vi "Wait for Operation Complete.vi"(8 "error in (no error)":errorcluster, 9 "Maximum Time (10000ms)":i32=10000, 11 "VISA resource name":refnum<visa-resource-name>) -> (0 "error out":errorcluster, 3 "VISA resource name out":refnum<visa-resource-name>)   [LabVIEW 2014, in "Agilent ESA PSA Series.lvlib"]
doc: "Waits for the current operation to finish. This VI should be called after Initiate VI.\n\n<B>Note:</B> \n\nUse this VI only with other low-level VIs. The high-level VIs automatically incorporate this functionality. This VI does not check the instrument status."
uses:
  Agilent ESA PSA Series.lvlib
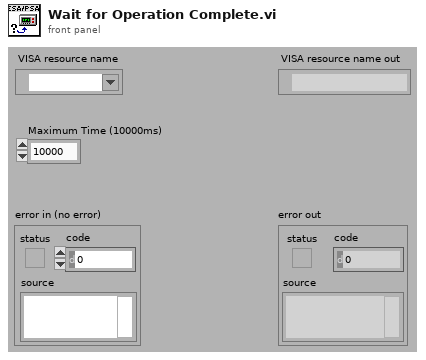
[diagram p1: front panel]
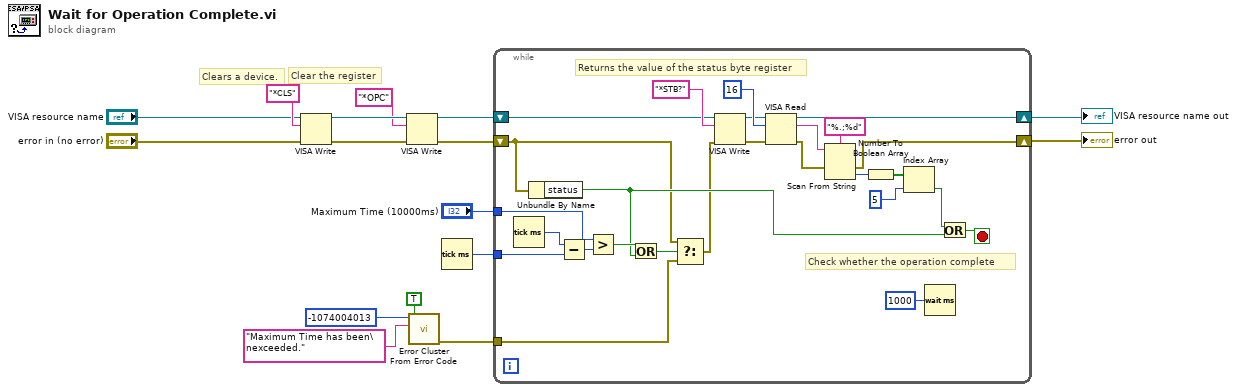
[diagram p0: block diagram]
diagram:
  # "Clears a device."
  # "Clear the register"
  n1 = VISA Write(VISA resource name="VISA resource name", write buffer="*CLS", error in (no error)="error in (no error)") -> (VISA resource name out=w6:refnum<visa-resource-name>, error out=w7:errorcluster)  [unwired: 1 out]
  n2 = VISA Write(VISA resource name=w6, write buffer="*OPC", error in (no error)=w7) -> (VISA resource name out=w5:refnum<visa-resource-name>, error out=w4:errorcluster)  [unwired: 1 out]
  n3 = call "Error Cluster From Error Code.vi"("show call chain? (False)"=TRUE, "error message (\"\")"="Maximum Time has been\nexceeded." ("error message (\"\")"), "error code (0)"=-1074004013) -> ("error out"=w10:errorcluster)  [unwired: 6 in]
  n4 = Tick Count (ms)() -> (millisecond timer value=w15:u32)
  n5 = while {
    tunnel: "Maximum Time (10000ms)" -> [w25]
    tunnel: w15 -> [w33]
    tunnel: w10 -> [w20]
    shift-right: [w31] -> w8
    shift-left: w4 -> [w18]
    shift-right: [w40] -> w9
    shift-left: w5 -> [w37]
    stop <- w26 stop-if-true
    # "Check whether the operation complete"
    # "Returns the value of the status byte register"
    n6 = Tick Count (ms)() -> (millisecond timer value=w34:u32)
    n7 = Unbundle By Name(w18) -> ("status"=w21:bool)
    n8 = Subtract(x=w34, y=w33) -> (x-y=w24:u32)
    n9 = Greater?(x=w25, y=w24) -> (0:w23:bool)
    n10 = Or(x=w23, y=w21) -> (x .or. y?=w22:bool)
    n11 = Select(t=w18, s=w22, f=w20) -> (s? t:f=w19:errorcluster)
    n12 = VISA Write(VISA resource name=w37, write buffer="*STB?", error in (no error)=w19) -> (VISA resource name out=w35:refnum<visa-resource-name>, error out=w36:errorcluster)  [unwired: 1 out]
    n13 = VISA Read(VISA resource name=w35, byte count=u32 16, error in (no error)=w36) -> (VISA resource name out=w40:refnum<visa-resource-name>, read buffer=w42:string, error out=w32:errorcluster)  [unwired: 1 out]
    n14 = Scan From String(format string="%.;%d", input string=w42, error in=w32) -> (error out=w31:errorcluster, output 1=w28:i32)  [unwired: 2 in, 2 out]
    n15 = Number To Boolean Array(number=w28) -> (Boolean array=w29:bool[])
    n16 = Index Array(array=w29, index=5) -> (element=w27:bool)
    n17 = Wait (ms)(milliseconds to wait=u32 1000) -> ()  [unwired: 1 out]
    n18 = Or(x=w27, y=w21) -> (x .or. y?=w26:bool)
  }
  "error out" <- w8
  "VISA resource name out" <- w9
